vi "Shutdown HW.vi"(8 "error in (no error)":errorcluster, 11 "Force Sensor in":refnum<class "Force Sensor.lvclass">) -> (0 "error out":errorcluster, 3 "Force Sensor out":refnum<class "Force Sensor.lvclass">)   [LabVIEW 2020, in "Force Sensor.lvclass"]
uses:
  Force Sensor.lvclass
  Sensor.lvclass
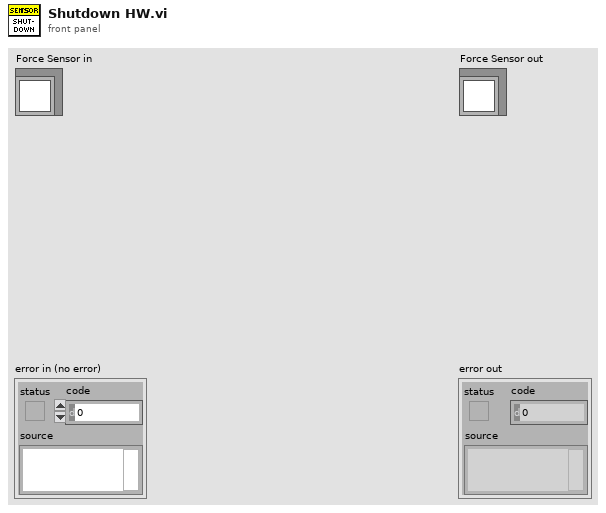
[diagram p1: front panel]
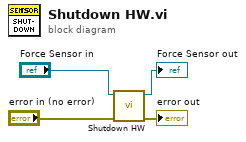
[diagram p0: block diagram]
diagram:
  n1 = call-parent "Shutdown HW.vi"("error in (no error)"="error in (no error)", "Sensor in"="Force Sensor in") -> ("error out"=→"error out":errorcluster, "Sensor out"=→"Force Sensor out":refnum<class "Force Sensor.lvclass">)  [unwired: 8 in]
